vi "Modifying the Color Table.vi"() -> ()   [LabVIEW 2018]
doc: "Demonstrates how to interactively and programmatically modify the color table for an intensity graph or intensity chart."
panel:
  in  "Update Marker Colors":bool
  in  "Custom Marker Colors":u32[](array[colorbox])=[16714752, 16748562, 16773418]
  in  "Stop":bool
  out "Intensity Graph":dbl[][](graph)
  # "Overview: Demonstrates how to interactively and programmatically modify the Color Table of an Intensity Graph or Intensity Chart.\nInstructions:\n1. Run the VI.\n2. Right-click one of the numbers on the Z Scale (the color ramp on the right side of the graph) and choose Marker Color to interactively change the color associated with that scale marker.  Observe the color change, and that the rest of the color ramp interpolates according to the new color.\n3. Click the Update Marker Colors button to programmatically apply new colors to the three markers on the Z Scale.\n4. Click Stop to stop the VI."
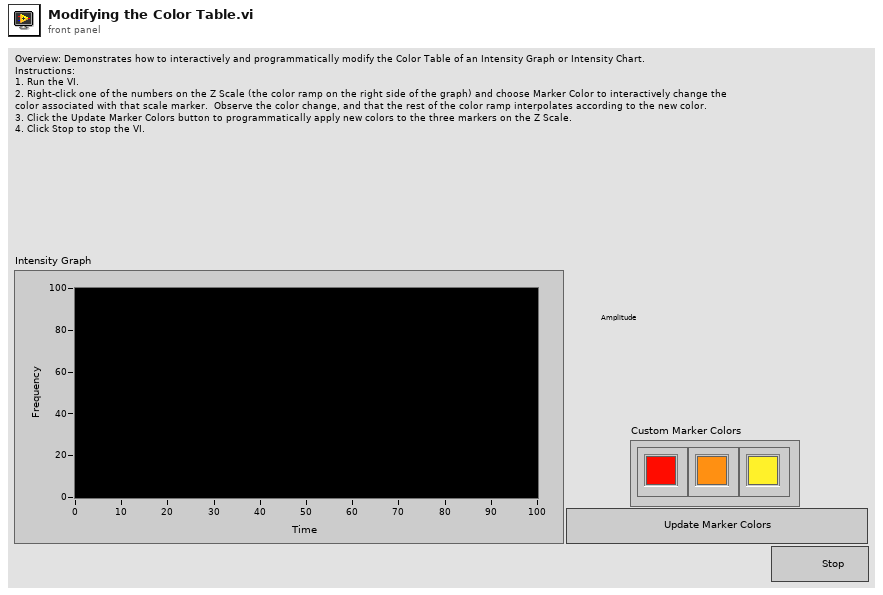
[diagram p1: front panel]
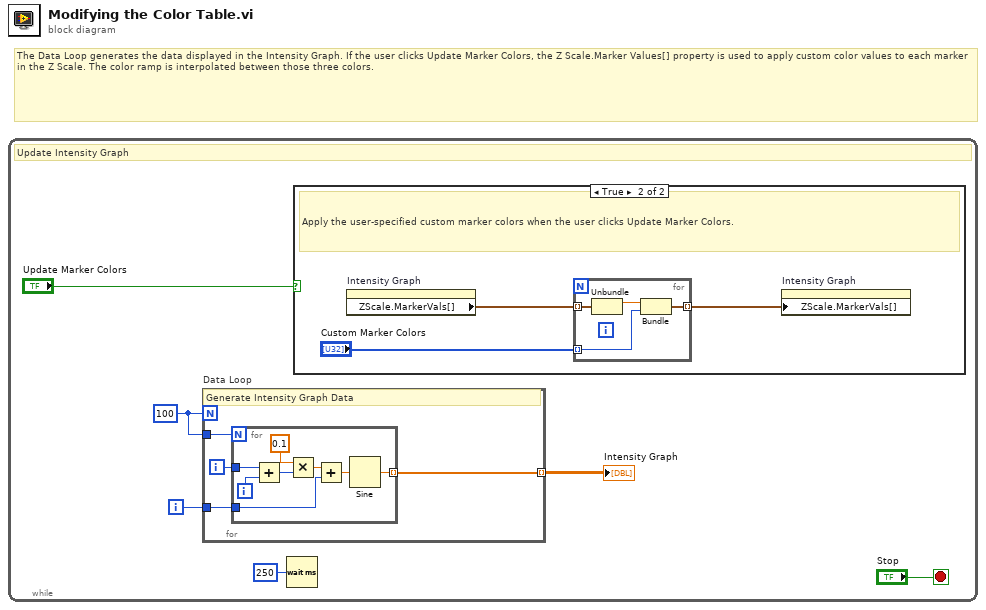
[diagram p0: block diagram]
diagram:
  # "The Data Loop generates the data displayed in the Intensity Graph. If the user clicks Update Marker Colors, the Z Scale.Marker Values[] property is used to apply custom color values to each marker in the Z Scale. The color ramp is interpolated between those three colors."
  n1 = while {
    i -> [w2]
    stop <- "Stop" stop-if-true
    w6 = 100
    # "Update Intensity Graph"
    n2 = for "Data Loop" {
      N: w6 -> [_]
      tunnel: [w17] -> w4 mode=indexing
      tunnel: w6 -> [w16]
      tunnel: w2 -> [w14]
      i -> [w15]
      # "Generate Intensity Graph Data"
      n3 = for {
        N: w16 -> [_]
        tunnel: [w25] -> w17 mode=indexing
        tunnel: w15 -> [w22]
        tunnel: w14 -> [w18]
        i -> [w23]
        n4 = Add(x=w22, y=w23) -> (x+y=w24:i32)
        n5 = Multiply(x=0.1, y=w24) -> (x*y=w21:dbl)
        n6 = Add(x=w21, y=w18) -> (x+y=w19:dbl)
        n7 = Sine(x=w19) -> (sin(x)=w25:dbl)
      }
    }
    "Intensity Graph" <- w4
    n8 = Wait (ms)(milliseconds to wait=u32 250) -> ()  [unwired: 1 out]
    n9 = case shown="True" "Update Marker Colors" {
      frame False {
        # "Do not manipulate the marker colors if the user has not pressed Update Marker Colors."
      }
      frame True {
        # "Apply the user-specified custom marker colors when the user clicks Update Marker Colors."
        n10 = property on="Intensity Graph" class="IntensityGraph (strict)"() -> ("ZScale.MarkerVals[]"=w9:cluster{dbl, u32}[])  [unwired: 2 in, 2 out]
        n11 = for {
          tunnel: w9 -> [w13] mode=indexing
          tunnel: "Custom Marker Colors" -> [w11] mode=indexing
          tunnel: [w10] -> w7 mode=indexing
          n12 = Unbundle(w13) -> (w12:dbl)  [unwired: 1 out]
          n13 = Bundle(w12, "Color Box"=w11) -> (w10:cluster{dbl, "Color Box":u32})  [unwired: 1 in]
        }
        n14 = property on="Intensity Graph" class="IntensityGraph (strict)"("ZScale.MarkerVals[]"=w7) -> ()  [unwired: 2 in, 2 out]
      }
    }
  }
